vi "Graph 4.vi"() -> ()   [LabVIEW 2024]
panel:
  out "XY Graph":cluster{"Array":dbl[], "Array 3":dbl[]}[](graph)
  in  "Array 3":dbl[](array[numeric])
  in  "Array 2":dbl[](array[numeric])
  in  "Array":dbl[](array[numeric])
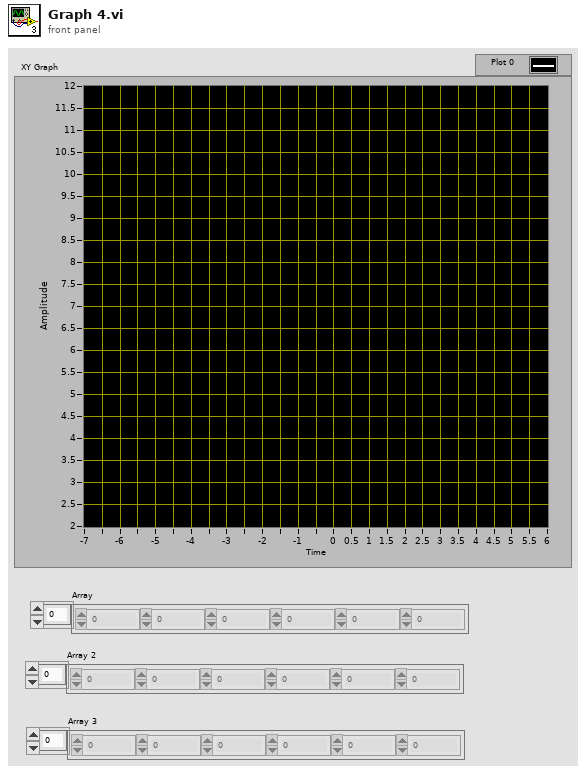
[diagram p1: front panel]
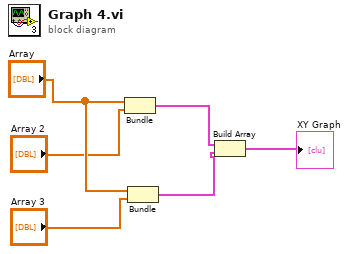
[diagram p0: block diagram]
diagram:
  n1 = Bundle("Array"="Array", "Array 2"="Array 2") -> (w3:cluster{"Array":dbl[], "Array 2":dbl[]})  [unwired: 1 in]
  n2 = Bundle("Array"="Array", "Array 3"="Array 3") -> (w2:cluster{"Array":dbl[], "Array 3":dbl[]})  [unwired: 1 in]
  n3 = Build Array(w3, w2) -> (→"XY Graph":cluster{"Array":dbl[], "Array 3":dbl[]}[])
